vi "Part 1.vi"(11 "Input":string) -> (3 "Output":i64)   [LabVIEW 2021]
uses:
  <userlib>/_OpenG.lib/string/string.llb/Convert EOLs (String)__ogtk.vi
  <vilib>/Analysis/NI_AAL_Geometry.lvlib
panel:
  in  "Input 2":string
  # "5189 too low"
  # "70354 too high"
  # "68115 correct"
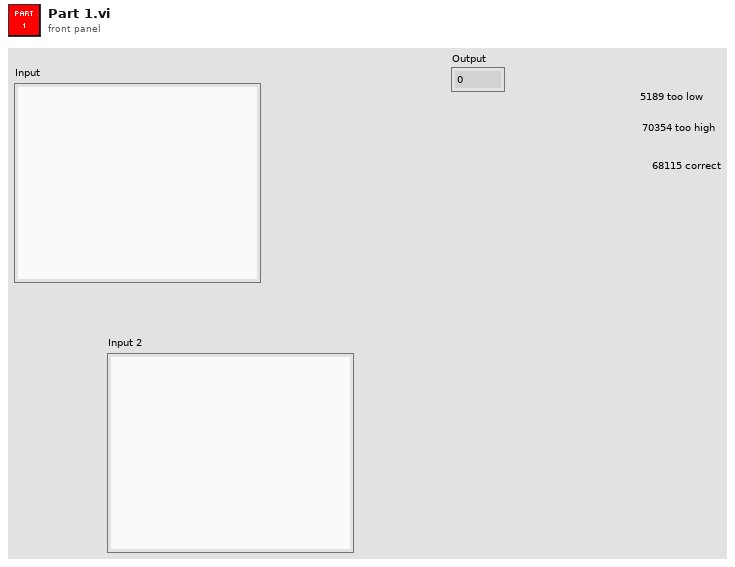
[diagram p1: front panel]
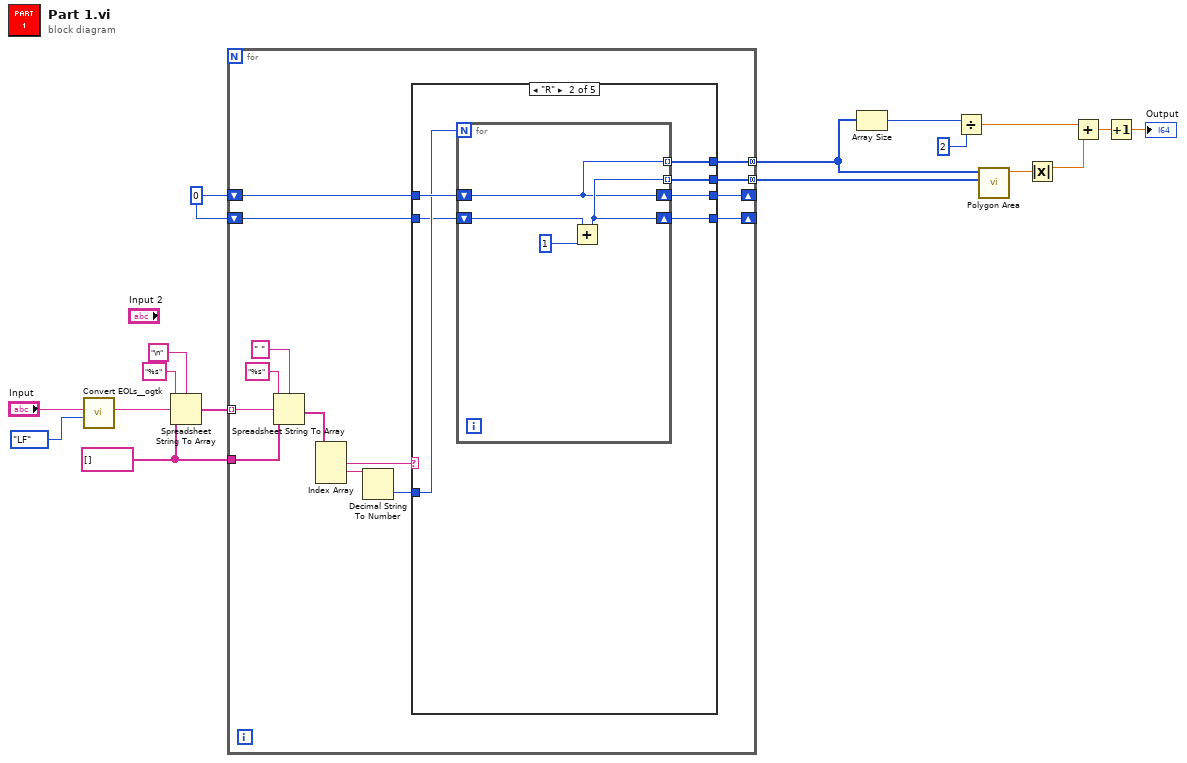
[diagram p0: block diagram]
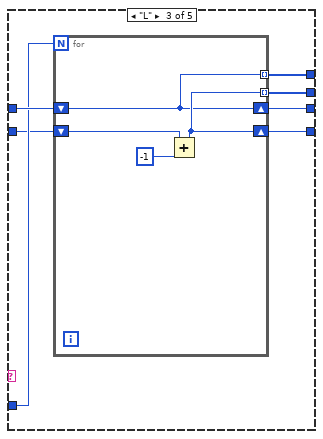
[diagram p3: hidden frame]
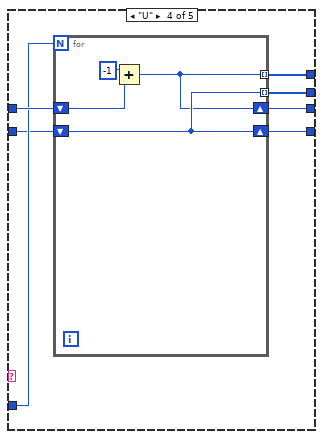
[diagram p4: hidden frame]
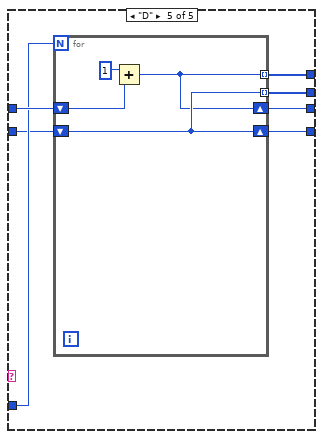
[diagram p5: hidden frame]
diagram:
  w5 = i64 0
  w11 = string[] []
  n1 = call-poly <userlib>:"Convert EOLs__ogtk.vi"("Convert to:"=enum16{"CR", "LF", "CRLF"}."LF", "String in"="Input") -> ("String out"=w14:string)  [unwired: 9 in]
  n2 = Spreadsheet String To Array(delimiter (Tab)="\n", format string="%s", spreadsheet string=w14, array type (2D Dbl)=w11) -> (array=w12:string[])
  n3 = for {
    tunnel: w12 -> [w30] mode=indexing
    tunnel: w11 -> [w29]
    shift-right: [w23] -> _
    shift-left: w5 -> [w24]
    tunnel: [w21] -> w4 mode=concatenating
    shift-right: [w19] -> _
    shift-left: w5 -> [w20]
    tunnel: [w18] -> w3 mode=concatenating
    n4 = Spreadsheet String To Array(delimiter (Tab)=" ", format string="%s", spreadsheet string=w30, array type (2D Dbl)=w29) -> (array=w27:string[])
    n5 = Index Array(array=w27) -> (element #1=w25:string, element #2=w26:string)  [unwired: 3 in, 1 out]
    n6 = Decimal String To Number(string=w26) -> (number=w22:i32)  [unwired: 2 in, 1 out]
    n7 = case shown="\"R\"" w25 {
      tunnel: w24 -> [w33 w40 w51 w62 w73]
      tunnel: [w33 w39 w50 w61 w72] -> w23
      tunnel: w22 -> [_ w38 w49 w60 w71]
      tunnel: [_ w37 w45 w56 w67] -> w21
      tunnel: w20 -> [w32 w36 w48 w59 w70]
      tunnel: [w32 w35 w47 w58 w69] -> w19
      tunnel: [_ w34 w46 w57 w68] -> w18
      frame Default {
      }
      frame "R" {
        n8 = for {
          N: w38 -> [_]
          shift-right: [w41] -> w39
          shift-left: w40 -> [w41]
          tunnel: [w42] -> w37 mode=indexing
          shift-right: [w42] -> w35
          shift-left: w36 -> [w43]
          tunnel: [w41] -> w34 mode=indexing
          n9 = Add(x=w43, y=i64 1) -> (x+y=w42:i64)
        }
      }
      frame "L" {
        n10 = for {
          N: w49 -> [_]
          shift-right: [w52] -> w50
          shift-left: w51 -> [w52]
          tunnel: [w53] -> w45 mode=indexing
          shift-right: [w53] -> w47
          shift-left: w48 -> [w54]
          tunnel: [w52] -> w46 mode=indexing
          n11 = Add(x=w54, y=i64 -1) -> (x+y=w53:i64)
        }
      }
      frame "U" {
        n12 = for {
          N: w60 -> [_]
          shift-right: [w63] -> w61
          shift-left: w62 -> [w64]
          tunnel: [w66] -> w56 mode=indexing
          shift-right: [w66] -> w58
          shift-left: w59 -> [w66]
          tunnel: [w63] -> w57 mode=indexing
          n13 = Add(x=i64 -1, y=w64) -> (x+y=w63:i64)
        }
      }
      frame "D" {
        n14 = for {
          N: w71 -> [_]
          shift-right: [w74] -> w72
          shift-left: w73 -> [w75]
          tunnel: [w77] -> w67 mode=indexing
          shift-right: [w77] -> w69
          shift-left: w70 -> [w77]
          tunnel: [w74] -> w68 mode=indexing
          n15 = Add(x=i64 1, y=w75) -> (x+y=w74:i64)
        }
      }
    }
  }
  n16 = Array Size(array=w3) -> (size(s)=w10:i32)
  n17 = Divide(x=w10, y=2) -> (x/y=w7:dbl)
  n18 = call <vilib>:"Polygon Area.vi"("Y"=w4, "X"=w3) -> ("signed area"=w9:dbl)  [unwired: 8 in, 1 out]
  n19 = Absolute Value(x=w9) -> (abs(x)=w8:dbl)
  n20 = Add(x=w7, y=w8) -> (x+y=w6:dbl)
  n21 = Increment(x=w6) -> (x+1=→"Output":dbl)
